vi "Run.vi"(8 "error in (no error)":errorcluster caption="entrée d'erreur (pas d'erreur)", 10 "X":string[][](array[string]), 11 "maxabs_scale.lvclass":refnum<class "maxabs_scale.lvclass">) -> (0 "error out":errorcluster caption="sortie d'erreur", 2 "Data":T1, 3 "maxabs_scale.lvclass":refnum<class "maxabs_scale.lvclass">)   [LabVIEW 2020, in "maxabs_scale.lvclass"]
uses:
  maxabs_scale.lvclass
  maxabs_scale.lvclass/maxabs_scale.ctl
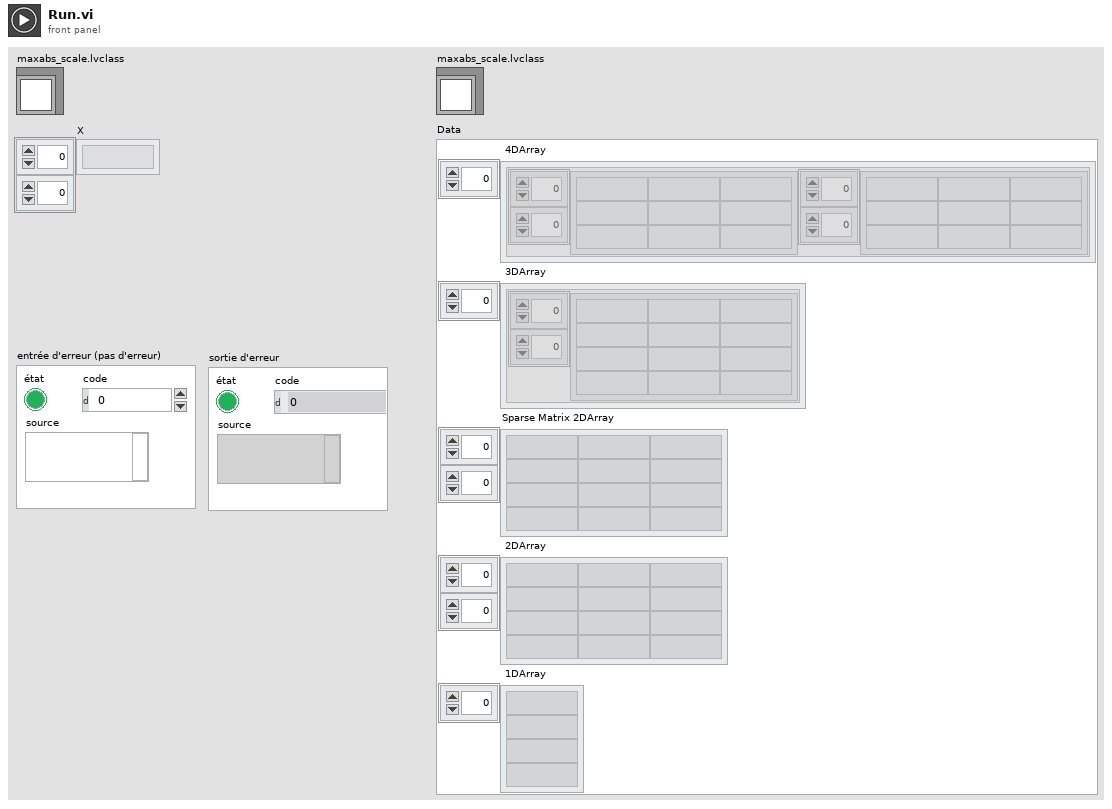
[diagram p1: front panel]
types:
  T1 = cluster{" 4DArray":cluster{"1":string[][], "2":string[][]}[], " 3DArray":cluster{"Tableau":string[][]}[], "Sparse Matrix 2DArray":string[][], " 2DArray":string[][], " 1DArray":string[]}
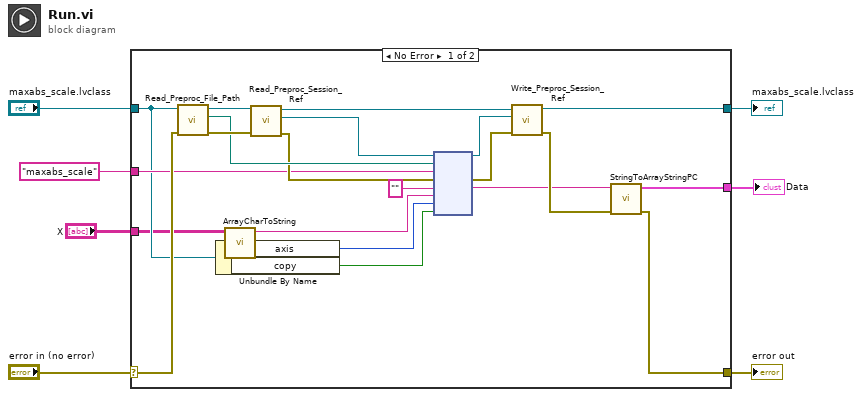
[diagram p0: block diagram]
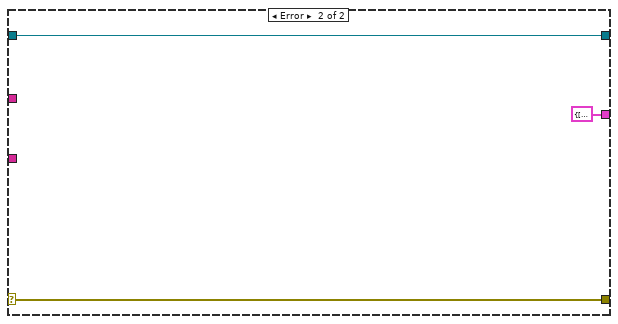
[diagram p2: hidden frame]
diagram:
  n1 = case shown="No Error" "error in (no error)" {
    selector: "error in (no error)" -> [w17 w31]
    tunnel: [w10 w31] -> w6
    tunnel: [w14 w30] -> w4
    tunnel: "maxabs_scale.lvclass" -> [w15 w30]
    tunnel: "maxabs_scale" ("Fonction") -> [w16 _]
    tunnel: [w11 T1 {" 4DArray"=[], " 3DArray"=[], "Sparse Matrix 2DArray"=[], " 2DArray"=[], " 1DArray"=[]} ("Data")] -> w1
    tunnel: "X" -> [w9 _]
    frame No Error {
      n2 = call-dynamic "Read_Preproc_File_Path.vi"("error in (no error)"=w17, "Python in"=w15) -> ("error out"=w27:errorcluster, "File_Path"=w24:path, "Python out"=w28:refnum<class "maxabs_scale.lvclass">)  [unwired: 7 in]
      n3 = Unbundle By Name(w15) -> ("axis"=w19:i32, "copy"=w18:bool)
      n4 = call "ArrayCharToString.vi"("TAB"=w9) -> ("Instruction"=w8:string)  [unwired: 10 in]
      n5 = call-dynamic "Read_Preproc_Session_Ref.vi"("error in (no error)"=w27, "Python in"=w28) -> ("error out"=w23:errorcluster, "Session_ref"=w25:refnum<k35>, "Python out"=w26:refnum<class "maxabs_scale.lvclass">)  [unwired: 7 in]
      n6 = node(w25, w24, w16, w23, "", w8, w19, w18) -> (w21:refnum<k35>, w22:errorcluster, w12:string)  [unwired: 3 in, 2 out]
      n7 = call-dynamic "Write_Preproc_Session_Ref.vi"("error in (no error)"=w22, "Session_ref"=w21, "Python in"=w26) -> ("error out"=w13:errorcluster, "Python out"=w14:refnum<class "maxabs_scale.lvclass">)  [unwired: 7 in]
      n8 = call "StringToArrayStringPC.vi"("sortie d'erreur"=w13, "Return value"=w12) -> ("sortie d'erreur"=w10:errorcluster, "Data"=w11:T1)  [unwired: 8 in]
    }
    frame Error {
    }
  }
  "error out" <- w6
  "maxabs_scale.lvclass" <- w4
  "Data" <- w1
